vi "fillColor.vi"() -> ()   [LabVIEW 2014]
panel:
  in  "Fill Color":u32 step=10
  out "Tank":dbl(slide) scale=0.0..10.0
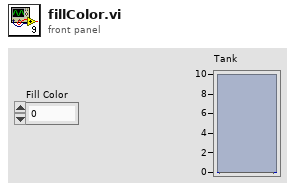
[diagram p1: front panel]
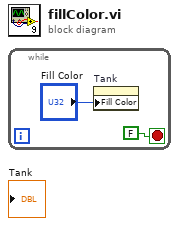
[diagram p0: block diagram]
diagram:
  n1 = while {
    stop <- FALSE stop-if-true
    n2 = property on="Tank" class="Slide (strict)"("Fill Color"="Fill Color") -> ()  [unwired: 2 in, 2 out]
  }
